vi "LCD Base Config.vi"(8 "error in (no error)":errorcluster, 9 "Rows":u8, 10 "Columns":u8, 11 "Arduino Resource in":T1) -> (0 "error out":errorcluster, 3 "Arduino Resource out":T1)   [LabVIEW 2011, in "LabVIEW Interface for Arduino.lvlib"]
doc: "Uses the default settings for the LCD screen. Clears and powers the screen, sets the cursor position to the top left corner, sets the direction as left-to-right, and sets the cursor as on and not blinking."
uses:
  LabVIEW Interface for Arduino.lvlib
  Private/Type Defs/Arduino Resource.ctl
  Private/Type Defs/Board Type.ctl
  Private/Type Defs/Direction.ctl
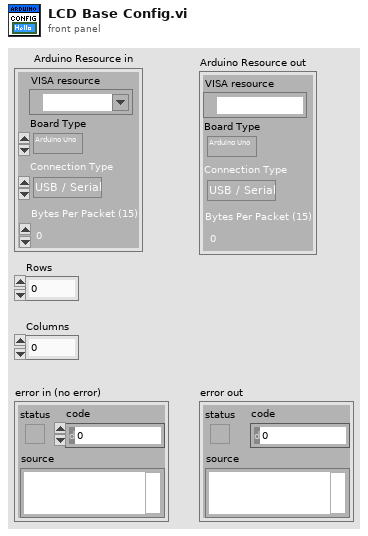
[diagram p1: front panel]
types:
  T1 = typedef "LabVIEW Interface for Arduino.lvlib/Arduino Resource.ctl" = cluster{"VISA resource":refnum<visa-resource-name>, "Board Type":T2, "Connection Type":enum8{"USB / Serial"}, "Bytes Per Packet (15)":u8}
  T2 = typedef "LabVIEW Interface for Arduino.lvlib/Board Type.ctl" = enum16{"Arduino Uno", "Dimuelanove w/Atmega 328", "Mega 2560", "Chipkit Uno32", "Chipkit Max32"}
  T3 = typedef "LabVIEW Interface for Arduino.lvlib/Direction.ctl" = enum8{"Left ", "Right"}
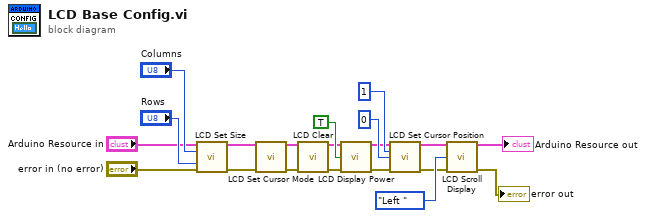
[diagram p0: block diagram]
diagram:
  n1 = call "LCD Set Size.vi"("Arduino Resource"="Arduino Resource in", "Columns"="Columns", "Rows"="Rows", "error in"="error in (no error)") -> ("Arduino Resource"=w5:T1, "error out"=w6:errorcluster)  [unwired: 10 in]
  n2 = call "LCD Set Cursor Mode.vi"("Arduino Resource"=w5, "error out"=w6) -> ("Arduino Resource"=w7:T1, "error out"=w8:errorcluster)  [unwired: 12 in]
  n3 = call "LCD Clear.vi"("Arduino Resource"=w7, "error in"=w8) -> ("Arduino Resource"=w9:T1, "error out"=w10:errorcluster)  [unwired: 12 in]
  n4 = call "LCD Display Power.vi"("Arduino Resource"=w9, "Display On? (T) 2"=TRUE, "error in"=w10) -> ("Arduino Resource"=w14:T1, "error out"=w15:errorcluster)  [unwired: 11 in]
  n5 = call "LCD Set Cursor Position.vi"("Arduino Resource"=w14, "Column"=u8 1, "Row"=u8 0, "error out"=w15) -> ("Arduino Resource"=w16:T1, "error out"=w17:errorcluster)  [unwired: 10 in]
  n6 = call "LCD Scroll Display.vi"("Arduino Resource"=w16, "Direction"=Direction."Left ", "error in"=w17) -> ("Arduino Resource"=→"Arduino Resource out":T1, "error out"=→"error out":errorcluster)  [unwired: 11 in]
